vi "Cleanup Panel.vi"(8 "error in (no error)":errorcluster, 10 "initial window state":T1(ring), 11 "vi reference in":refnum<vi>) -> (0 "error out":errorcluster, 3 "vi reference out":refnum<vi>)   [LabVIEW 2019, in "MicronGRPCGeneratedServer.lvlib"]
uses:
  MicronGRPCGeneratedServer.lvlib
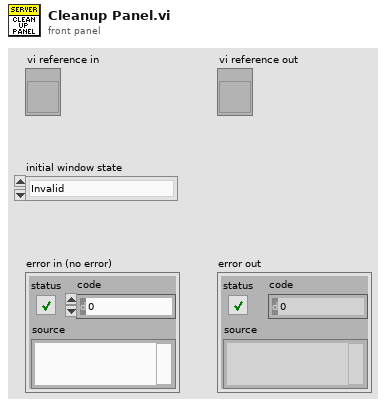
[diagram p1: front panel]
types:
  T1 = enum32{"Invalid", "Standard", "Closed", "Hidden", "Minimized", "Maximized"}
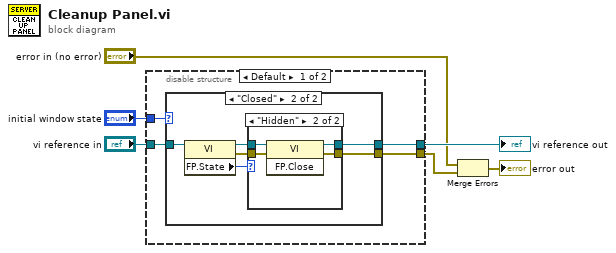
[diagram p0: block diagram]
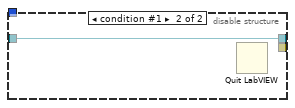
[diagram p4: hidden frame]
diagram:
  n1 = disable-structure shown="Default" {
    disable-tunnel: "vi reference in" -> [w10 w24]
    disable-tunnel: [w9 w24] -> w5
    disable-tunnel: [w8 _] -> w2
    disable-tunnel: "initial window state" -> [w7 _]
    frame condition #0 (active) {
      n2 = case shown="\"Closed\"" w7 {
        tunnel: w10 -> [w11 w15]
        tunnel: [w11 w17] -> w9
        tunnel: [_ w16] -> w8
        frame Default {
        }
        frame "Closed" {
          n3 = property class="VI"(reference=w15) -> (reference out=w14:refnum<vi>, error out=w13:errorcluster, "FP.State"=w12:T1)  [unwired: 1 in]
          n4 = case shown="\"Hidden\"" w12 {
            tunnel: [w19 w23] -> w17
            tunnel: [w18 w22] -> w16
            tunnel: w14 -> [w19 w21]
            tunnel: w13 -> [w18 w20]
            frame Default {
            }
            frame "Hidden" {
              n5 = invoke class="VI" method="FP.Close"(reference=w21, error in=w20) -> (reference out=w23:refnum<vi>, error out=w22:errorcluster)  [unwired: 1 in, 1 out]
            }
          }
        }
      }
    }
    frame condition #1 {
      n6 = Quit LabVIEW() -> ()  [unwired: 1 in]
    }
  }
  "vi reference out" <- w5
  n7 = Merge Errors("error in (no error)", w2) -> (→"error out":errorcluster)
